vi "SimpleSerial.vi"() -> ()   [LabVIEW 2021]
doc: "This example performs a serial port write and a serial port read. The parameters set for the serial port must match the parameters of the connected instrument or device. The VISA Configure Serial Port VI sets the configuration parameters. The front panel displays the controls used to configure the basic parameters, such as baud rate, data bits, and parity. The VI passes the VISA resource name to other VIs that perform operations on that VISA resource. The VISA Write function sends a command to the serial device and the VISA Read function returns data based on the command. The VISA Close function then closes the reference to the serial device. It is important to close the reference; otherwise, further communication through that port might not be possible."
uses:
  <vilib>/Instr/_visa.llb/VISA Configure Serial Port (Instr).vi
panel:
  in  "flow control":u16(ring) items=["None"=0, "XON/XOFF"=1, "RTS/CTS"=2, "DTR/DSR"=4]
  in  "stop bits":u16(ring)=10 items=["1.0"=10, "1.5"=15, "2.0"=20]
  in  "parity":u16(ring) items=["None", "Odd", "Even", "Mark", "Space"]
  in  "data bits":u16=8 min=5 max=8 step=1
  in  "baud rate":u32=9600
  in  "Command":string="*IDN?\n"
  out "bytes read":u32
  in  "delay before read (ms)":u32=500
  out "Response":string
  in  "VISA resource name":refnum<visa-resource-name>="COM1"
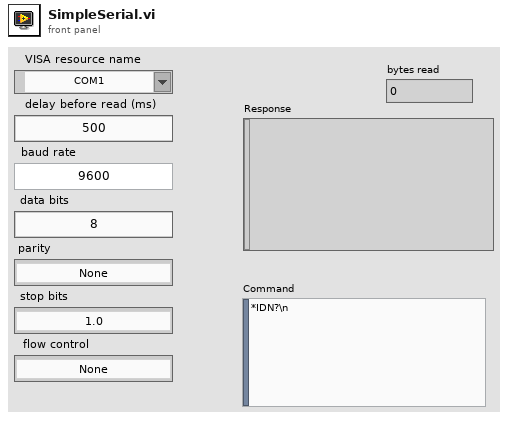
[diagram p1: front panel]
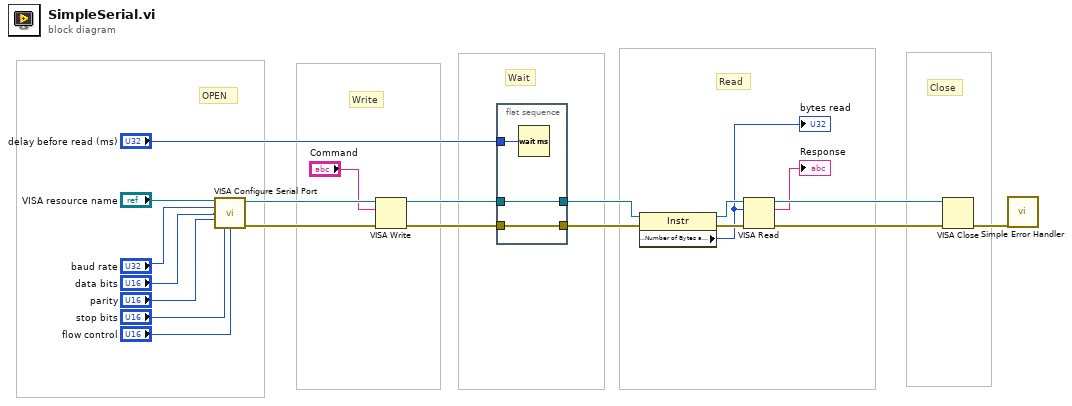
[diagram p0: block diagram]
diagram:
  # "Close"
  # "Read"
  # "Wait"
  # "Write"
  # "OPEN"
  n1 = call-poly "VISA Configure Serial Port"("VISA resource name"="VISA resource name", "baud rate (9600)"="baud rate", "data bits (8)"="data bits", "parity (0:none)"="parity", "stop bits (10: 1 bit)"="stop bits", "flow control (0:none)"="flow control") -> ("VISA resource name out"=w19:refnum<visa-resource-name>, "error out"=w20:errorcluster)  [unwired: 3 in, 5 out]
  n2 = VISA Write(VISA resource name=w19, write buffer="Command", error in (no error)=w20) -> (VISA resource name out=w13:refnum<visa-resource-name>, error out=w15:errorcluster)  [unwired: 1 out]
  n3 = flat-sequence {
    tunnel: w15 -> [w23]
    tunnel: [w23] -> w14
    tunnel: w13 -> [w22]
    tunnel: [w22] -> w12
    tunnel: "delay before read (ms)" -> [w24]
    frame #0 {
      n4 = Wait (ms)(milliseconds to wait=w24) -> ()  [unwired: 1 out]
    }
  }
  n5 = property class="Instr"(reference=w12, error in=w14) -> (reference out=w9:refnum<visa-resource-name>, error out=w8:errorcluster, "Serial Settings:Number of Bytes at Serial Port"=w6:u32)
  "bytes read" <- w6
  n6 = VISA Read(VISA resource name=w9, byte count=w6, error in (no error)=w8) -> (VISA resource name out=w17:refnum<visa-resource-name>, read buffer=→"Response":string, error out=w18:errorcluster)  [unwired: 1 out]
  n7 = VISA Close(VISA resource name=w17, error in (no error)=w18) -> (error out=w16:errorcluster)
  n8 = call <vilib>:"Simple Error Handler.vi"("error in (no error)"=w16) -> ()  [unwired: 1 in, 8 out]
